vi "HOST_laser_SEL.vi"() -> ()   [LabVIEW 2018]
uses:
  <vilib>/userdefined/High Color/nirio_resource_hc.ctl
  <vilib>/FPGAPlugInAG/PXI-7841R/niLvFpga_Open_PXI-7841R.vi
  <vilib>/rvi/interface/common/dynamic/niFpgaDynamicAddResources.vi
  <vilib>/FPGAPlugInAG/Dynamic/niLvFpga_Reset_Dynamic.vi
  <vilib>/FPGAPlugInAG/Dynamic/niLvFpga_Run_Dynamic.vi
  <vilib>/Utility/error.llb/Error Cluster From Error Code.vi
  <vilib>/rvi/errors/niLvFpgaAdjustHostInterfaceError.vi
  <vilib>/FPGAPlugInAG/Dynamic/niLvFpga_Close_Dynamic.vi
  <vilib>/rvi/interface/nirviOpenFPGA/nirviOpenFPGA.xnode
  FPGA Bitfiles/iCLNGNQI_FPGATarget_Target_OrC3no1FGAk.lvbitx
  <vilib>/rvi/interface/nirviMethod/nirviMethod.xnode
  <vilib>/rvi/interface/nirviReadWriteControl/nirviReadWriteControl.xnode
  <vilib>/rvi/interface/nirviCloseFPGA/nirviCloseFPGA.xnode
  NiFpgaLv.dll
  <vilib>/rvi/interface/Simulation/niFpgaSimulationCallBeginRW.vi
panel:
  in  "Стоп":bool
  out "NSIN":i16
  out "NCOS":i16
  out "PCOS":i16
  out "PSIN":i16
  in  "resource name":T1="PXI1Slot6"
  out "Waveform Chart":cluster{dbl, dbl, dbl, dbl}(graph)={-0.294189453125, -0.3173828125, -0.3009033203125, -0.313720703125}
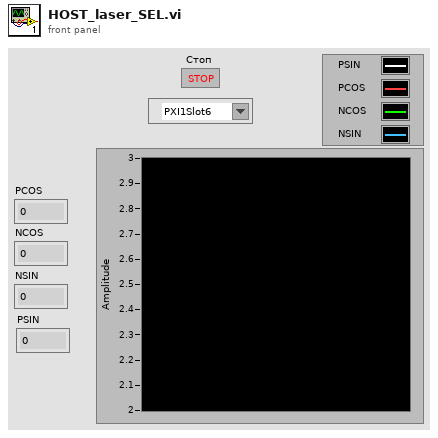
[diagram p1: front panel]
types:
  T1 = typedef "nirio_resource_hc.ctl" = tag
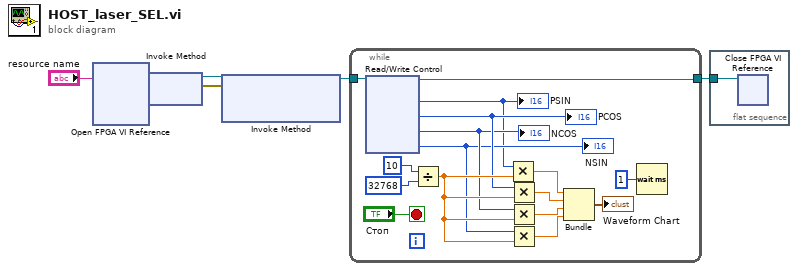
[diagram p0: block diagram]
diagram:
  n1 = xnode "Open FPGA VI Reference"("resource name"="resource name") -> ("FPGA VI Reference Out"=w2:refnum<k20>, "error out"=w4:errorcluster)  [unwired: 1 in]
  n2 = xnode "Invoke Method"("FPGA VI Reference In"=w2, "error in"=w4) -> ("FPGA VI Reference Out"=w5:refnum<k20>, "error out"=w3:errorcluster)
  n3 = xnode "Invoke Method"("FPGA VI Reference In"=w5, "error in"=w3) -> ("FPGA VI Reference Out"=w1:refnum<k20>)  [unwired: 1 in, 1 out]
  n4 = while {
    tunnel: [w10] -> w7
    tunnel: w1 -> [w9]
    stop <- "Стоп" stop-if-true
    n5 = xnode "Read/Write Control"("FPGA VI Reference In"=w9) -> ("FPGA VI Reference Out"=w10:refnum<k20>, "PSIN"=w11:i16, "PCOS"=w14:i16, "NCOS"=w13:i16, "NSIN"=w12:i16)  [unwired: 1 in, 1 out]
    "PSIN" <- w11
    "PCOS" <- w14
    "NCOS" <- w13
    "NSIN" <- w12
    n6 = Divide(x=10, y=32768) -> (x/y=w20:dbl)
    n7 = Multiply(x=w11, y=w20) -> (x*y=w19:dbl)
    n8 = Multiply(x=w14, y=w20) -> (x*y=w18:dbl)
    n9 = Multiply(x=w13, y=w20) -> (x*y=w17:dbl)
    n10 = Multiply(x=w12, y=w20) -> (x*y=w16:dbl)
    n11 = Bundle(w19, w18, w17, w16) -> (→"Waveform Chart":cluster{dbl, dbl, dbl, dbl})  [unwired: 1 in]
    n12 = Wait (ms)(milliseconds to wait=u32 1) -> ()  [unwired: 1 out]
  }
  n13 = flat-sequence {
    tunnel: w7 -> [w24]
    frame #0 {
      n14 = xnode "Close FPGA VI Reference"("FPGA VI Reference In"=w24) -> ()  [unwired: 1 in, 1 out]
    }
  }
